vi "Set Trigger Style.vi"(8 "error in (no error)":errorcluster, 11 "style":u32) -> (0 "error out":errorcluster)   [LabVIEW 2021, in "vmmso.lvlib"]
doc: "DLL_API void WINAPI SetTriggerStyle(unsigned int style);"
uses:
  vmmso.lvlib
  vmmso.dll
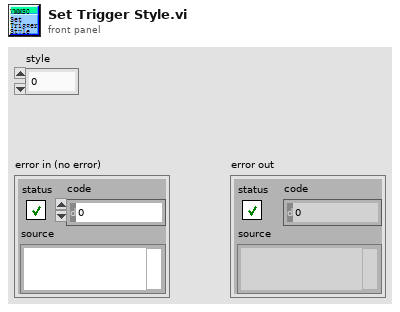
[diagram p1: front panel]
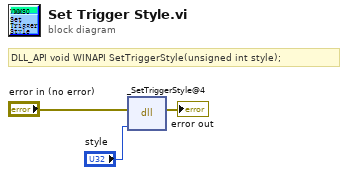
[diagram p0: block diagram]
diagram:
  # "DLL_API void WINAPI SetTriggerStyle(unsigned int style);"
  n1 = dll-call lib="O:/MSO/library/demo-Labview/vmmso/vmmso.*" fn="_SetTriggerStyle@4"(error in="error in (no error)", "style"="style") -> (error out=→"error out":errorcluster)  [unwired: 4 in, 1 out]
